vi "PrintInOutNakTransactions.vi"(7 "Path":path=path "C:/LabViewTesty", 9 "Colors":u32[](array[colorbox])=[65535, 16711935, 16776960, 16770816, 11796658, 4210752], 10 "Trasaction In-Out-Nak":string[](array[string]), 11 "Pie Chart Transactions:\n In - Out- Nak":picture) -> ()   [LabVIEW 2014]
panel:
  out "Transactions In Out Nak":T1={"Pie Chart Transactions:\n In - Out- Nak"=bytes[270], "Date"="", "Time"="", "Colors"=[65535, 16711935, 16776960, 16770816, 11796658, 4210752], "Trasaction In-Out-Nak"=[]}
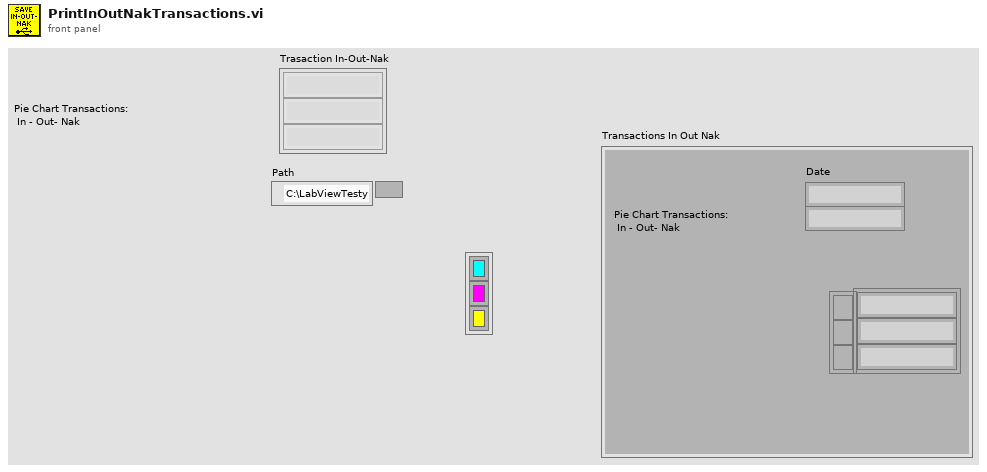
[diagram p1: front panel]
types:
  T1 = cluster{"Pie Chart Transactions:\n In - Out- Nak":picture, "Date":string, "Time":string, "Colors":u32[], "Trasaction In-Out-Nak":string[]}
  T2 = typedef "imagedata.ctl" = cluster{"image type":i32, "image depth":i32, "image":u8[], "mask":u8[], "colors":u32[], "Rectangle":cluster{"left":i16, "top":i16, "right":i16, "bottom":i16}}
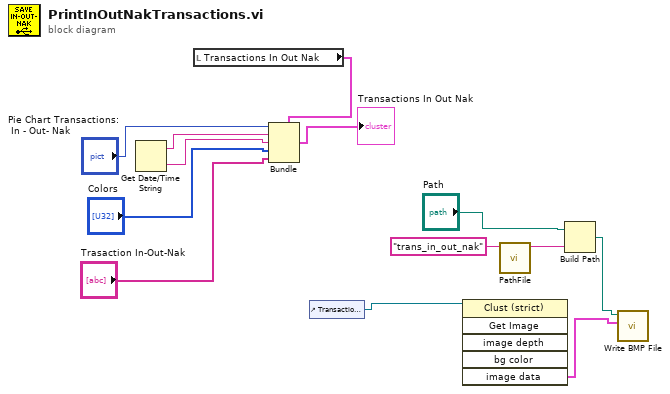
[diagram p0: block diagram]
diagram:
  n1 = Get Date/Time String() -> (date string=w9:string, time string=w8:string)  [unwired: 3 in]
  n2 = local read "Transactions In Out Nak"() -> (w13:T1)
  n3 = Bundle(cluster=w13, "Pie Chart Transactions:\n In - Out- Nak"="Pie Chart Transactions:\n In - Out- Nak", "Date"=w9, "Time"=w8, "Colors"="Colors", "Trasaction In-Out-Nak"="Trasaction In-Out-Nak") -> (→"Transactions In Out Nak":T1)
  n4 = control-ref of="Transactions In Out Nak"() -> (w1:refnum<vi>)
  n5 = invoke class="Clust (strict)" method="Get Image"(reference=w1) -> ("image data"=w6:T2)  [unwired: 5 in, 5 out]
  n6 = call "PathFile.vi"("NameFile"="trans_in_out_nak") -> ("stringNameFile"=w2:string)  [unwired: 10 in]
  n7 = Build Path(base path="Path", name or relative path=w2) -> (appended path=w5:path)
  n8 = call <vilib>:"Write BMP File.vi"("image data"=w6, "path to BMP file"=w5) -> ()  [unwired: 8 in, 2 out]
